vi "Get GUIDs for Month.vi"(8 "error in (no error)":errorcluster, 10 "Month Timestamp":timestamp=timestamp(3819510000 s since 1904-01-01) format="%<%x>T", 11 "Time Entry-INI in":refnum<class "Time Entry-INI.lvclass">) -> (0 "error out":errorcluster, 2 "GUIDs for Month":string[](array[string]), 3 "Time Entry-INI out":refnum<class "Time Entry-INI.lvclass">)   [LabVIEW 2020, in "Time Entry-INI.lvclass"]
uses:
  Time Entry-INI.lvclass
  Time Entry-INI.lvclass/Time Entry-INI.ctl
  <vilib>/Utility/config.llb/NI_LVConfig.lvlib
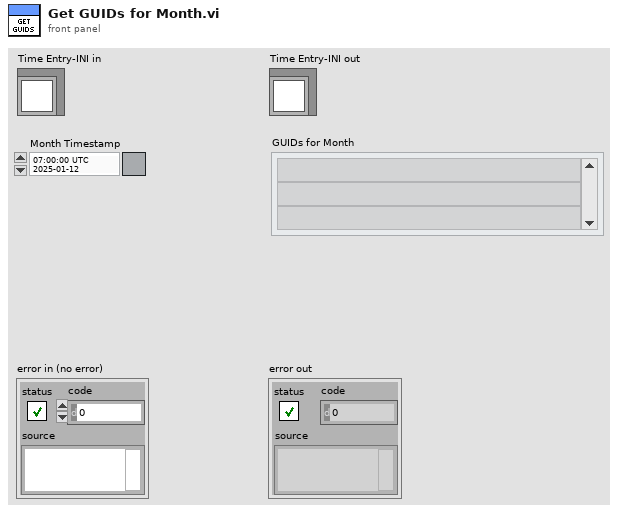
[diagram p1: front panel]
types:
  T1 = typedef "LVDateTimeRec.ctl" = cluster{"fractional second":dbl, "second":i32, "minute":i32, "hour":i32, "day of month":i32, "month":i32, "year":i32, "day of week":i32, "day of year":i32, "DST":i32}
  T2 = typedef "NI_LVConfig.lvlib/Config Data RefNum.ctl" = refnum<k1>
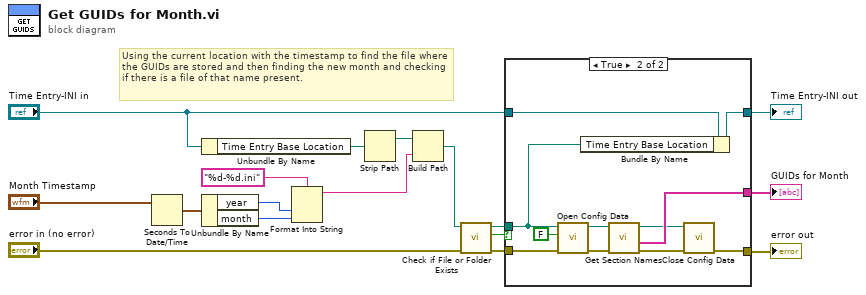
[diagram p0: block diagram]
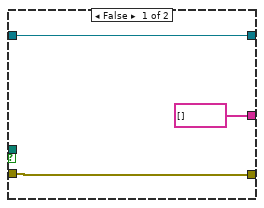
[diagram p2: hidden frame]
diagram:
  # "Using the current location with the timestamp to find the file where the GUIDs are stored and then finding the new month and checking if there is a file of that name present."
  n1 = Seconds To Date/Time(time stamp (now)="Month Timestamp") -> (date time rec=w16:T1)  [unwired: 1 in]
  n2 = Unbundle By Name("Time Entry-INI in") -> ("Time Entry Base Location"=w12:path)
  n3 = Unbundle By Name(w16) -> ("year"=w14:i32, "month"=w13:i32)
  n4 = Format Into String(format string="%d-%d.ini" ("time format string (%c)"), w14, w13) -> (resulting string=w10:string)  [unwired: 2 in, 1 out]
  n5 = Strip Path(path=w12) -> (stripped path=w11:path)  [unwired: 1 out]
  n6 = Build Path(base path=w11, name or relative path=w10) -> (appended path=w9:path)
  n7 = call <vilib>:"Check if File or Folder Exists.vi"("error in (no error)"="error in (no error)", "path"=w9) -> ("error out"=w6:errorcluster, "file or folder exists?"=w3:bool, "dup path"=w7:path)  [unwired: 7 in]
  n8 = case shown="True" w3 {
    tunnel: w7 -> [_ w21]
    tunnel: w6 -> [w20 w31]
    tunnel: [w20 w24] -> w5
    tunnel: [string[] [] ("GUIDs for Month") w27] -> w4
    tunnel: "Time Entry-INI in" -> [w18 w23]
    tunnel: [w18 w22] -> w1
    frame False {
    }
    frame True {
      n9 = call <vilib>:"Open Config Data.vi"("error in (no error)"=w31, "create file if necessary (T)"=FALSE, "configuration file path"=w21) -> ("error out"=w28:errorcluster, "refnum"=w29:T2)  [unwired: 6 in, 1 out]
      n10 = Bundle By Name(cluster=w23, "Time Entry Base Location"=w21) -> (w22:refnum<class "Time Entry-INI.lvclass">)
      n11 = call <vilib>:"Get Section Names.vi"("error in (no error)"=w28, "refnum"=w29) -> ("error out"=w25:errorcluster, "section names"=w27:string[], "refnum out"=w26:T2)  [unwired: 7 in]
      n12 = call <vilib>:"Close Config Data.vi"("error in (no error)"=w25, "refnum"=w26) -> ("error out"=w24:errorcluster)  [unwired: 8 in, 1 out]
    }
  }
  "error out" <- w5
  "Time Entry-INI out" <- w1
  "GUIDs for Month" <- w4
